vi "isPath.vi"(8 "error in TCP":errorcluster, 10 "string Path in":string, 11 "connection ID in":refnum<k5>) -> (0 "error out TCP":errorcluster, 1 "Path is Ok?":bool, 2 "absolute path":path, 3 "connection ID out":refnum<k5>)   [LabVIEW 2010]
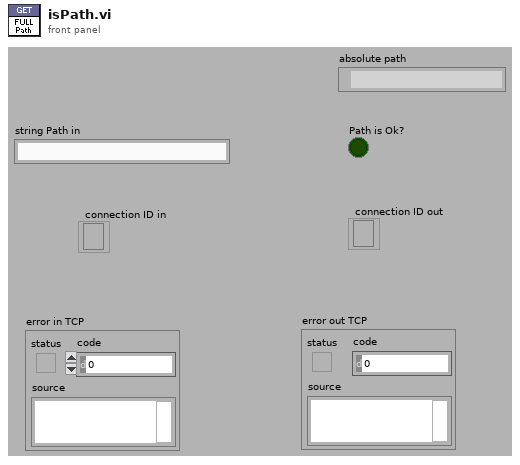
[diagram p1: front panel]
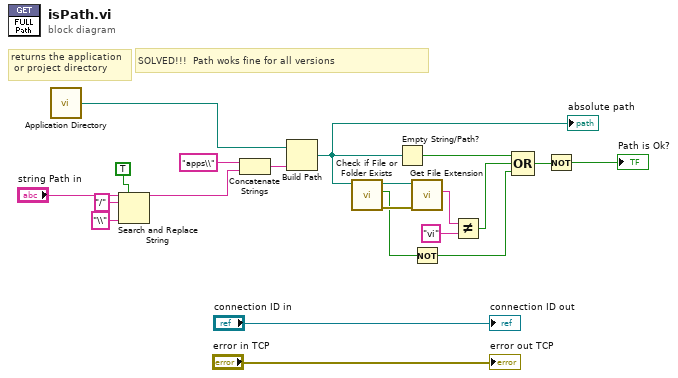
[diagram p0: block diagram]
diagram:
  # "returns the application\n or project directory"
  # "SOLVED!!!  Path woks fine for all versions"
  n1 = call <vilib>:"Application Directory.vi"() -> ("Application Directory"=w1:path)
  n2 = Search and Replace String(replace all?=TRUE ("replace all? (F)"), input string="string Path in", search string="/", replace string="\\" ("replace string (\"\")")) -> (result string=w5:string)  [unwired: 1 in, 6 out]
  n3 = Concatenate Strings("apps\\" ("string"), w5) -> (w21:string)
  n4 = Build Path(base path=w1, name or relative path=w21) -> (appended path=w12:path)
  "absolute path" <- w12
  n5 = call <vilib>:"Check if File or Folder Exists.vi"("path"=w12) -> ("error out"=w18:errorcluster, "file or folder exists?"=w14:bool, "dup path"=w19:path)  [unwired: 1 in, 7 out]
  n6 = Empty String/Path?(string/path=w12) -> (empty?=w16:bool)
  n7 = call <vilib>:"Get File Extension.vi"("error in (no error)"=w18, "file"=w19) -> ("lowercase file extension"=w2:string)  [unwired: 9 out]
  n8 = Not(x=w14) -> (.not. x?=w13:bool)
  n9 = Not Equal?(x=w2, y="vi") -> (x != y?=w15:bool)
  n10 = Compound Arithmetic op=OR(w16, w15, w13) -> (w4:bool)
  n11 = Not(x=w4) -> (.not. x?=→"Path is Ok?":bool)
  "connection ID out" <- "connection ID in"
  "error out TCP" <- "error in TCP"
